vi "Get Series CFG.vi"(11 "Series Actor in":refnum<class "Series Actor.lvclass">) -> (2 "Series CFG":string, 3 "Series Actor out":refnum<class "Series Actor.lvclass">)   [LabVIEW 2024, in "Series Actor.lvlib" / "Series Actor.lvclass"]
uses:
  Series Actor.lvclass
  Series Actor.lvclass/Series Actor.ctl
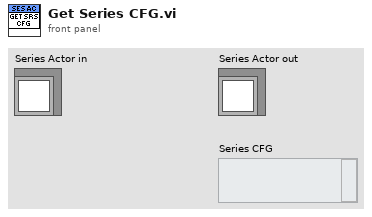
[diagram p1: front panel]
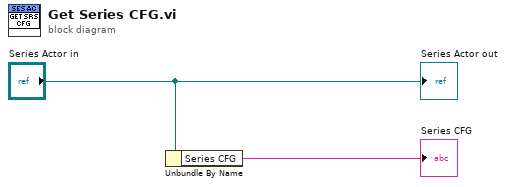
[diagram p0: block diagram]
diagram:
  n1 = Unbundle By Name("Series Actor in") -> ("Series CFG"=→"Series CFG":string)
  "Series Actor out" <- "Series Actor in"
